vi "Guess A Number.vi"() -> ()   [LabVIEW 2016]
panel:
  in  "Cancel Button":bool
  out "Random":dbl
  out "100":dbl
  out "0":dbl
  in  "OK Button":bool
  in  "User":dbl
  # "GUESS THE NUMBER"
  # "?"
  # "PLEASE INSERT YOUR VALUE HERE"
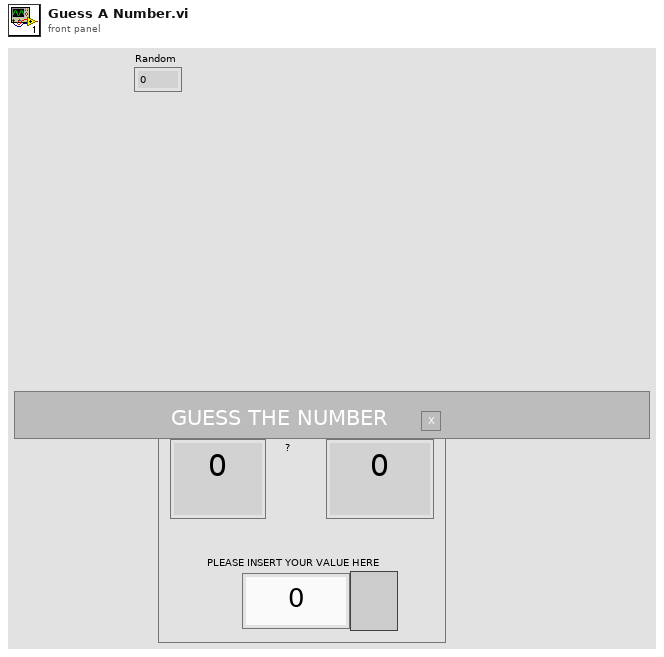
[diagram p1: front panel]
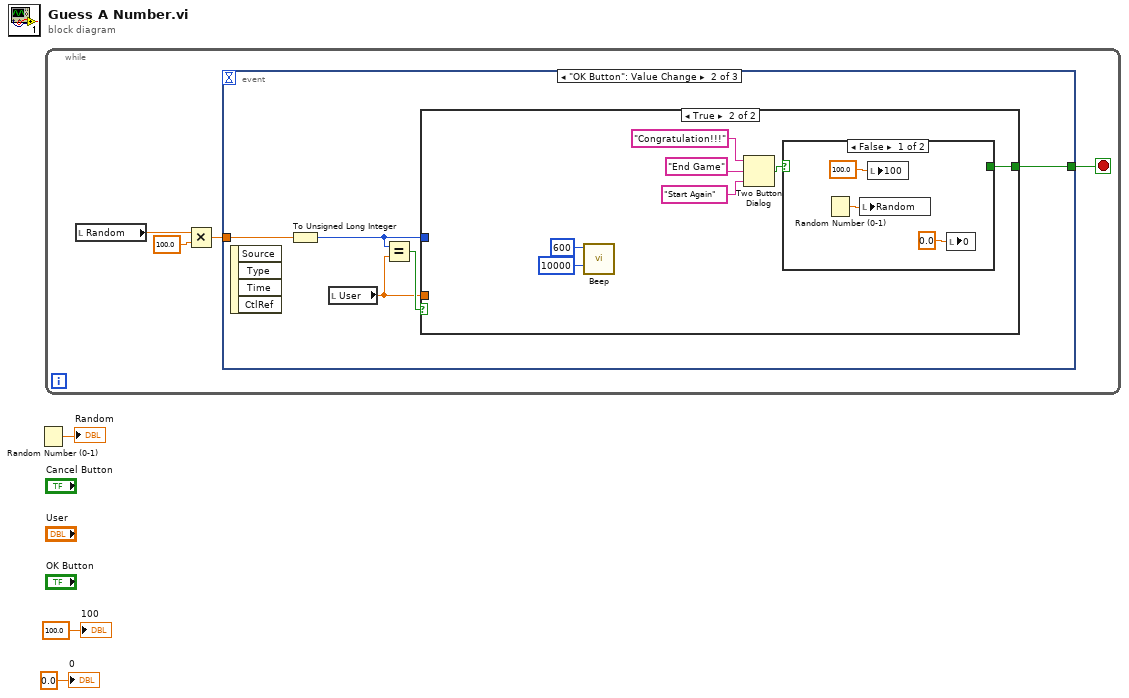
[diagram p0: block diagram]
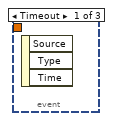
[diagram p2: hidden frame]
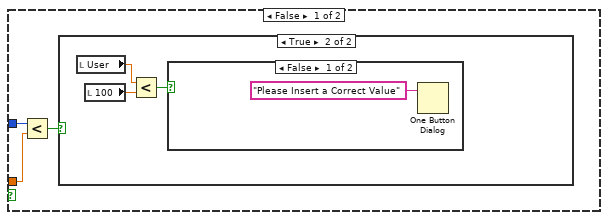
[diagram p3: hidden frame]
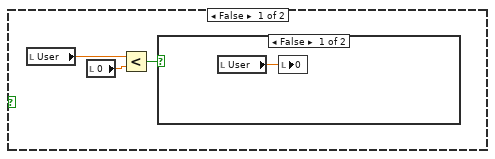
[diagram p4: hidden frame]
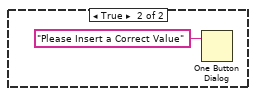
[diagram p5: hidden frame]
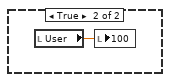
[diagram p6: hidden frame]
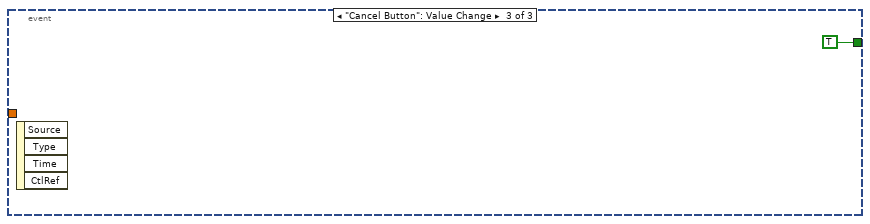
[diagram p8: hidden frame]
diagram:
  n1 = Random Number (0-1)() -> (number: 0 to 1=→"Random":dbl)
  n2 = while {
    stop <- w7 stop-if-true
    n3 = local read "Random"() -> (w4:dbl)
    n4 = Multiply(x=w4, y=100.0) -> (x*y=w5:dbl)
    n5 = event shown="[1] \"OK Button\": Value Change" {
      selector: _ -> [_ _ _]
      dyn-events: _ -> [_ _ _]
      timeout: _ -> [_ _ _]
      tunnel: w5 -> [_ w12 _]
      tunnel: [_ w8 TRUE] -> w7
      event Timeout {
        n6 = event-data() -> ()  [unwired: 1 in, 3 out]
      }
      event "OK Button": Value Change {
        n7 = event-data() -> ()  [unwired: 1 in, 4 out]
        n8 = To Unsigned Long Integer(number=w12) -> (unsigned 32bit integer=w9:u32)
        n9 = local read "User"() -> (w10:dbl)
        n10 = Equal?(x=w9, y=w10) -> (x = y?=w11:bool)
        n11 = case shown="True" w11 {
          tunnel: w10 -> [w14 _]
          tunnel: w9 -> [w15 _]
          tunnel: [_ w28] -> w8
          frame False {
            n12 = Less?(x=w15, y=w14) -> (x < y?=w13:bool)
            n13 = case shown="True" w13 {
              frame False {
                n14 = local read "User"() -> (w17:dbl)
                n15 = local read "0"() -> (w18:dbl)
                n16 = Less?(x=w17, y=w18) -> (x < y?=w16:bool)
                n17 = case shown="False" w16 {
                  frame False {
                    n18 = local read "User"() -> (w19:dbl)
                    n19 = local write "0"(w19) -> ()
                  }
                  frame True {
                    n20 = One Button Dialog(message="Please Insert a Correct Value") -> ()  [unwired: 1 in, 1 out]
                  }
                }
              }
              frame True {
                n21 = local read "User"() -> (w23:dbl)
                n22 = local read "100"() -> (w22:dbl)
                n23 = Less?(x=w23, y=w22) -> (x < y?=w21:bool)
                n24 = case shown="False" w21 {
                  frame False {
                    n25 = One Button Dialog(message="Please Insert a Correct Value") -> ()  [unwired: 1 in, 1 out]
                  }
                  frame True {
                    n26 = local read "User"() -> (w25:dbl)
                    n27 = local write "100"(w25) -> ()
                  }
                }
              }
            }
          }
          frame True {
            n28 = call <vilib>:"Beep.vi"("duration (msec)"=u32 10000, "frequency (Hz)"=u32 600) -> ()  [unwired: 10 in]
            n29 = Two Button Dialog(message="Congratulation!!!", 1:"Start Again" ("F button name (\"Cancel\")"), 2:"End Game" ("T button name (\"OK\")")) -> (T button?=w29:bool)
            n30 = case shown="False" w29 {
              selector: w29 -> [_ w36]
              tunnel: [_ w36] -> w28
              frame False {
                n31 = Random Number (0-1)() -> (number: 0 to 1=w33:dbl)
                n32 = local write "Random"(w33) -> ()
                n33 = local write "100"(100.0 ("100")) -> ()
                n34 = local write "0"(0.0 ("0")) -> ()
              }
              frame True {
              }
            }
          }
        }
      }
      event "Cancel Button": Value Change {
        n35 = event-data() -> ()  [unwired: 1 in, 4 out]
      }
    }
  }
  "0" <- 0.0 ("0")
  "100" <- 100.0 ("100")
